vi "s-lab第2章 布尔型数据1-6.vi"() -> ()   [LabVIEW 2013]
panel:
  in  "停止 2":bool
  out "报警灯":bool
  out "报警液位":dbl
  out "当前液位":dbl
  out "液罐":dbl(slide) scale=0.0..10.0
  in  "进水管 2":dbl(slide) scale=0.0..10.0
  in  "出水管":dbl(slide) scale=0.0..10.0
  in  "进水管 1":dbl(slide) scale=0.0..10.0
  in  "停止":bool
  out "数值 9":dbl
  out "灯 2":bool
  out "灯 1":bool
  in  "数值 8":dbl
  in  "数值 7":dbl
  out "布尔 3":bool
  out "数值 6":dbl
  out "数值 5":dbl
  out "布尔 2":bool
  in  "数值 4":dbl
  in  "数值 3":dbl
  out "布尔":bool
  in  "数值 2":dbl
  in  "数值":dbl
  out "指示灯 2":bool
  out "指示灯 1":bool
  in  "开关 2":bool
  in  "开关 1":bool
  # "例 1"
  # "例 4"
  # "例 5"
  # "例 2"
  # "例 6"
  # "例 3"
  # "书上答案错误"
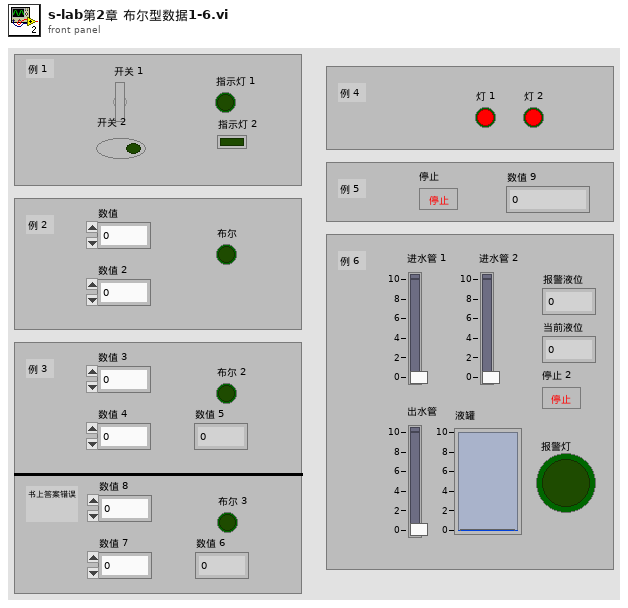
[diagram p1: front panel]
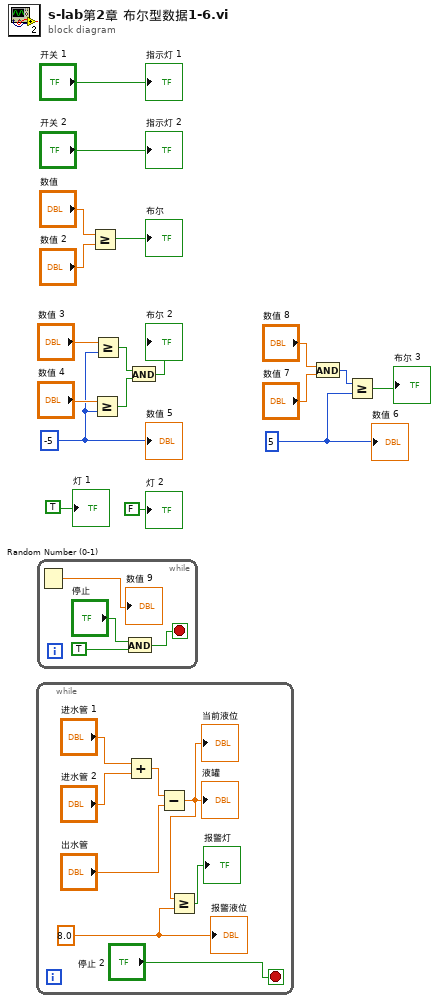
[diagram p0: block diagram]
diagram:
  w4 = 5
  w11 = -5
  n1 = while {
    stop <- "停止 2" stop-if-true
    w25 = 8.0
    n2 = Add(x="进水管 1", y="进水管 2") -> (x+y=w22:dbl)
    n3 = Subtract(x=w22, y="出水管") -> (x-y=w26:dbl)
    "液罐" <- w26
    "当前液位" <- w26
    n4 = Greater Or Equal?(x=w26, y=w25) -> (x >= y?=→"报警灯":bool)
    "报警液位" <- w25
  }
  n5 = while {
    stop <- w27 stop-if-true
    n6 = Random Number (0-1)() -> (number: 0 to 1=→"数值 9":dbl)
    n7 = And(x="停止", y=TRUE) -> (x .and. y?=w27:bool)
  }
  n8 = Greater Or Equal?(x="数值", y="数值 2") -> (x >= y?=→"布尔":bool)
  n9 = Greater Or Equal?(x="数值 4", y=w11) -> (x >= y?=w8:bool)
  n10 = Greater Or Equal?(x="数值 3", y=w11) -> (x >= y?=w9:bool)
  n11 = And(x=w9, y=w8) -> (x .and. y?=→"布尔 2":bool)
  n12 = And(x="数值 8", y="数值 7") -> (x .and. y?=w5:i32)
  n13 = Greater Or Equal?(x=w5, y=w4) -> (x >= y?=→"布尔 3":bool)
  "指示灯 1" <- "开关 1"
  "指示灯 2" <- "开关 2"
  "数值 5" <- w11
  "数值 6" <- w4
  "灯 1" <- TRUE
  "灯 2" <- FALSE
